vi "Text Format Definition Dialog.vi"(8 "Error In":errorcluster) -> (0 "Error Out":errorcluster, 1 "Result":T1, 2 "Theme Name":string, 3 "Notebook Theme":T2 {"[Named Text Styles]"."Text Formatting"."Font Size" min=6.0 step=1.0})   [LabVIEW 2021, in "Notebook.lvlib"]
doc: "Define text format for different styles"
uses:
  Notebook.lvlib
  Rich Text Box/Text Format List.ctl
  Rich Text Box/Text Colors.ctl
  Notebook Theme.ctl
  Rich Text Box/Named Text Style.ctl
  Rich Text Box/Text Formatting.ctl
  Rich Text Box/Text Style.ctl
  Rich Text Box/Text Alignment.ctl
  Notebook Theme Edit Result.ctl
  Notebook Parameters List.ctl
  Variant/Variant to Data/Variant to String.vi
  Rich Text Box/Rich Text Box.lvlib
  System.Windows.Forms
  Variant/Variant to Data/Variant to Data.lvlib
panel:
  in  "Close":bool
  in  "Mark for Deletion":bool
  in  "Theme Name":string
  in  "Use Font Size for all Styles":bool
  in  "Use Alignment for all Styles":bool
  in  "Use Style for all Styles":bool
  in  "Use Background Color for all Styles":bool
  in  "Use Text Color for all Styles":bool
  in  "Use Font for all Styles":bool
  in  "Cancel":bool
  in  "Apply":bool
  in  "Page Color":T5=enum."White"
  in  "Text Style":T8
  in  "Example Content":refnum<k24>(container) caption="Text Example"
  in  "Text Formatting":T9={"Font"=0, "Text Color"=enum."Unchanged", "Background Color"=enum."Unchanged", "Style"=enum."Regular", "Font Size"=6.0, "Alignment"=enum."Left"} {"Font Size" min=6.0 step=1.0; "Font" items=["Adobe Devanagari", "Agency FB", "Algerian", "Arial", "Arial Black", "Arial Narrow", "Arial Rounded MT Bold", "Bahnschrift", "Bahnschrift Condensed", "Bahnschrift Light", "Bahnschrift Light Condensed", "Bahnschrift Light SemiCondensed", "Bahnschrift SemiBold", "Bahnschrift SemiBold Condensed", "Bahnschrift SemiBold SemiConden", "Bahnschrift SemiCondensed", "Bahnschrift SemiLight", "Bahnschrift SemiLight Condensed", "Bahnschrift SemiLight SemiConde", "Barlow Condensed", "Barlow Condensed Black", "Barlow Condensed ExtraBold", "Barlow Condensed ExtraLight", "Barlow Condensed Light", "Barlow Condensed Medium", "Barlow Condensed SemiBold", "Barlow Condensed Thin", "Baskerville Old Face", "Bauhaus 93", "Bell MT", "Berlin Sans FB", "Berlin Sans FB Demi", "Bernard MT Condensed", "Blackadder ITC", "Bodoni MT", "Bodoni MT Black", "Bodoni MT Condensed", "Bodoni MT Poster Compressed", "Book Antiqua", "Bookman Old Style", "Bookshelf Symbol 7", "Bradley Hand ITC", "Britannic Bold", "Broadway", "Brush Script MT", "Calibri", "Calibri Light", "Californian FB", "Calisto MT", "Cambria", "Cambria Math", "Candara", "Candara Light", "Cascadia Code", "Cascadia Code ExtraLight", "Cascadia Code Light", "Cascadia Code SemiBold", "Cascadia Code SemiLight", "Cascadia Mono", "Cascadia Mono ExtraLight", "Cascadia Mono Light", "Cascadia Mono SemiBold", "Cascadia Mono SemiLight", "Castellar", "Caveat", "Centaur", "Century", "Century Gothic", "Century Schoolbook", "Chiller", "Colonna MT", "Comic Sans MS", "Consolas", "Constantia", "Cooper Black", "Copperplate Gothic Bold", "Copperplate Gothic Light", "Corbel", "Corbel Light", "Cormorant Infant", "Cormorant Infant Light", "Cormorant Infant Medium", "Cormorant Infant SemiBold", "Courier New", "Curlz MT", "Dosis", "Dubai", "Dubai Light", "Dubai Medium", "Ebrima", "Edwardian Script ITC", "Elephant", "Engravers MT", "Eras Bold ITC", "Eras Demi ITC", "Eras Light ITC", "Eras Medium ITC", "Euclid", "Euclid Extra", "Euclid Fraktur", "Euclid Math One", "Euclid Math Two", "Euclid Symbol", "Felix Titling", "Fences", "Footlight MT Light", "Forte", "Franklin Gothic Book", "Franklin Gothic Demi", "Franklin Gothic Demi Cond", "Franklin Gothic Heavy", "Franklin Gothic Medium", "Franklin Gothic Medium Cond", "Freestyle Script", "French Script MT", "Gabriola", "Gadugi", "Garamond", "Georgia", "Gigi", "Gill Sans MT", "Gill Sans MT Condensed", "Gill Sans MT Ext Condensed Bold", "Gill Sans Ultra Bold", "Gill Sans Ultra Bold Condensed", "Gloucester MT Extra Condensed", "Goudy Old Style", "Goudy Stout", "Haettenschweiler", "Harlow Solid Italic", "Harrington", "High Tower Text", "HoloLens MDL2 Assets", "HYSWLongFangSong", "Impact", "Imprint MT Shadow", "Informal Roman", "Ink Free", "Javanese Text", "Jokerman", "Juice ITC", "Kristen ITC", "Kunstler Script", "Lato", "Lato Black", "Lato Hairline", "Lato Light", "Leelawadee", "Leelawadee UI", "Leelawadee UI Semilight", "Lucida Bright", "Lucida Calligraphy", "Lucida Console", "Lucida Fax", "Lucida Handwriting", "Lucida Sans", "Lucida Sans Typewriter", "Lucida Sans Unicode", "Magneto", "Maiandra GD", "Malgun Gothic", "Malgun Gothic Semilight", "Marlett", "Matura MT Script Capitals", "Microsoft Himalaya", "Microsoft JhengHei", "Microsoft JhengHei Light", "Microsoft JhengHei UI", "Microsoft JhengHei UI Light", "Microsoft New Tai Lue", "Microsoft PhagsPa", "Microsoft Sans Serif", "Microsoft Tai Le", "Microsoft Uighur", "Microsoft YaHei", "Microsoft YaHei Light", "Microsoft YaHei UI", "Microsoft YaHei UI Light", "Microsoft Yi Baiti", "MingLiU-ExtB", "MingLiU_HKSCS-ExtB", "Mistral", "Modern No. 20", "Mongolian Baiti", "Monotype Corsiva", "Montserrat", "Montserrat Black", "Montserrat ExtraBold", "Montserrat ExtraLight", "Montserrat Light", "Montserrat Medium", "Montserrat SemiBold", "Montserrat Thin", "MS Gothic", "MS Outlook", "MS PGothic", "MS Reference Sans Serif", "MS Reference Specialty", "MS UI Gothic", "MT Extra", "MT Extra Tiger", "MV Boli", "Myanmar Text", "Niagara Engraved", "Niagara Solid", "Nirmala UI", "Nirmala UI Semilight", "Noto Sans", "Noto Serif", "NSimSun", "OCR A Extended", "Old English Text MT", "Onyx", "Open Sans", "Open Sans ExtraBold", "Open Sans Light", "Open Sans SemiBold", "Origin", "Oswald", "Oswald ExtraLight", "Oswald Light", "Oswald Medium", "Oswald SemiBold", "Palace Script MT", "Palatino Linotype", "Papyrus", "Parchment", "Perpetua", "Perpetua Titling MT", "Playbill", "PMingLiU-ExtB", "Poor Richard", "Pristina", "Rage Italic", "Raleway", "Raleway Black", "Raleway ExtraBold", "Raleway ExtraLight", "Raleway Light", "Raleway Medium", "Raleway SemiBold", "Raleway Thin", "Ravie", "Roboto", "Roboto Black", "Roboto Condensed", "Roboto Condensed Light", "Roboto Light", "Roboto Medium", "Roboto Slab", "Roboto Slab Black", "Roboto Slab Light", "Roboto Slab Medium", "Roboto Slab Thin", "Roboto Thin", "Rockwell", "Rockwell Condensed", "Rockwell Extra Bold", "Script MT Bold", "Segoe MDL2 Assets", "Segoe Print", "Segoe Script", "Segoe UI", "Segoe UI Black", "Segoe UI Emoji", "Segoe UI Historic", "Segoe UI Light", "Segoe UI Semibold", "Segoe UI Semilight", "Segoe UI Symbol", "Showcard Gothic", "SimSun", "SimSun-ExtB", "SimSun-ExtG", "Sitka Banner", "Sitka Display", "Sitka Heading", "Sitka Small", "Sitka Subheading", "Sitka Text", "Snap ITC", "Source Code Pro", "Source Code Pro Black", "Source Code Pro ExtraLight", "Source Code Pro Light", "Source Code Pro Semibold", "Source Sans Pro", "Source Sans Pro Black", "Source Sans Pro ExtraLight", "Source Sans Pro Light", "Source Sans Pro SemiBold", "Stencil", "Sylfaen", "Symbol", "Symbol Tiger", "Symbol Tiger Expert", "Tahoma", "Tempus Sans ITC", "Tiger", "Tiger Expert", "Times New Roman", "Trebuchet MS", "Tw Cen MT", "Tw Cen MT Condensed", "Tw Cen MT Condensed Extra Bold", "Univers-CondBoldOblique", "Univers-Condensed", "Univers-CondensedBold", "UniversCond", "UniversCondBold", "UniversCondLight", "UniversCondLightOblique", "UniversCondOblique", "Verdana", "Viner Hand ITC", "Vivaldi", "Vladimir Script", "Webdings", "Wide Latin", "Wingdings", "Wingdings 2", "Wingdings 3", "Yu Gothic", "Yu Gothic Light", "Yu Gothic Medium", "Yu Gothic UI", "Yu Gothic UI Light", "Yu Gothic UI Semibold", "Yu Gothic UI Semilight", "Zilla Slab", "Zilla Slab Light", "Zilla Slab Medium", "Zilla Slab SemiBold", "ZWAdobeF"]}
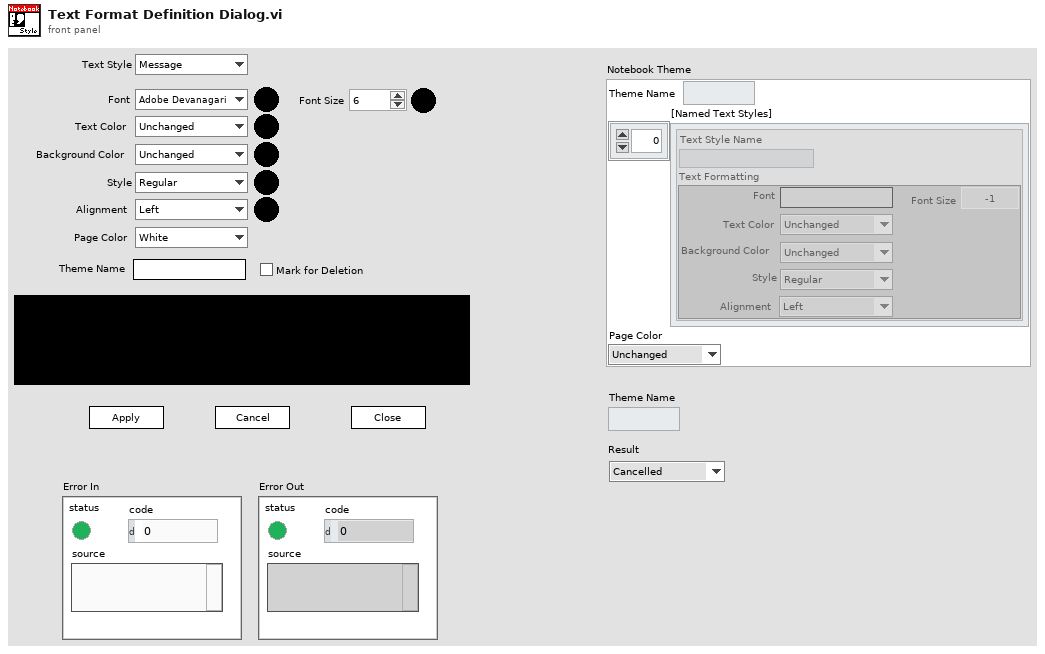
[diagram p1: front panel]
types:
  T1 = typedef "Notebook.lvlib/Notebook Theme Edit Result.ctl" = enum16{"Cancelled", "Modified Theme", "New Theme", "Remove Theme"}
  T2 = typedef "Notebook.lvlib/Notebook Theme.ctl" = cluster{"Theme Name":string, "[Named Text Styles]":T3[], "Page Color":T5}
  T3 = typedef "Notebook.lvlib/Named Text Style.ctl" = cluster{"Text Formatting":T4, "Text Style Name":string}
  T4 = typedef "Rich Text Box.lvlib/Text Formatting.ctl" = cluster{"Font":string, "Text Color":T5, "Background Color":T5, "Style":T6, "Font Size":dbl, "Alignment":T7}
  T5 = typedef "Rich Text Box.lvlib/Text Colors.ctl" = enum16{"Unchanged", "Black", "Blue", "Cyan", "Maroon", "Gray", "Violet", "Green", "Light Green", "Orange", "Yellow", "Magenta", "Red", "White"}
  T6 = typedef "Rich Text Box.lvlib/Text Style.ctl" = enum16{"Regular", "Bold", "Italic", "Underline", "Strikeout"}
  T7 = typedef "Rich Text Box.lvlib/Text Alignment.ctl" = enum16{"Left", "Right", "Center"}
  T8 = typedef "Notebook.lvlib/Text Format List.ctl" = enum16{"Message", "Result", "Error", "Setting", "Verbose", "Warning"}
  T9 = cluster{"Font":u16, "Text Color":T5, "Background Color":T5, "Style":T6, "Font Size":dbl, "Alignment":T7}
  T10 = typedef "Notebook.lvlib/Notebook Parameters List.ctl" = enum16{"First Opening?", "Saved Notebook?", "Saved Notebook Path", "Beep on Error?", "Notebook Themes", "Current Theme Name"}
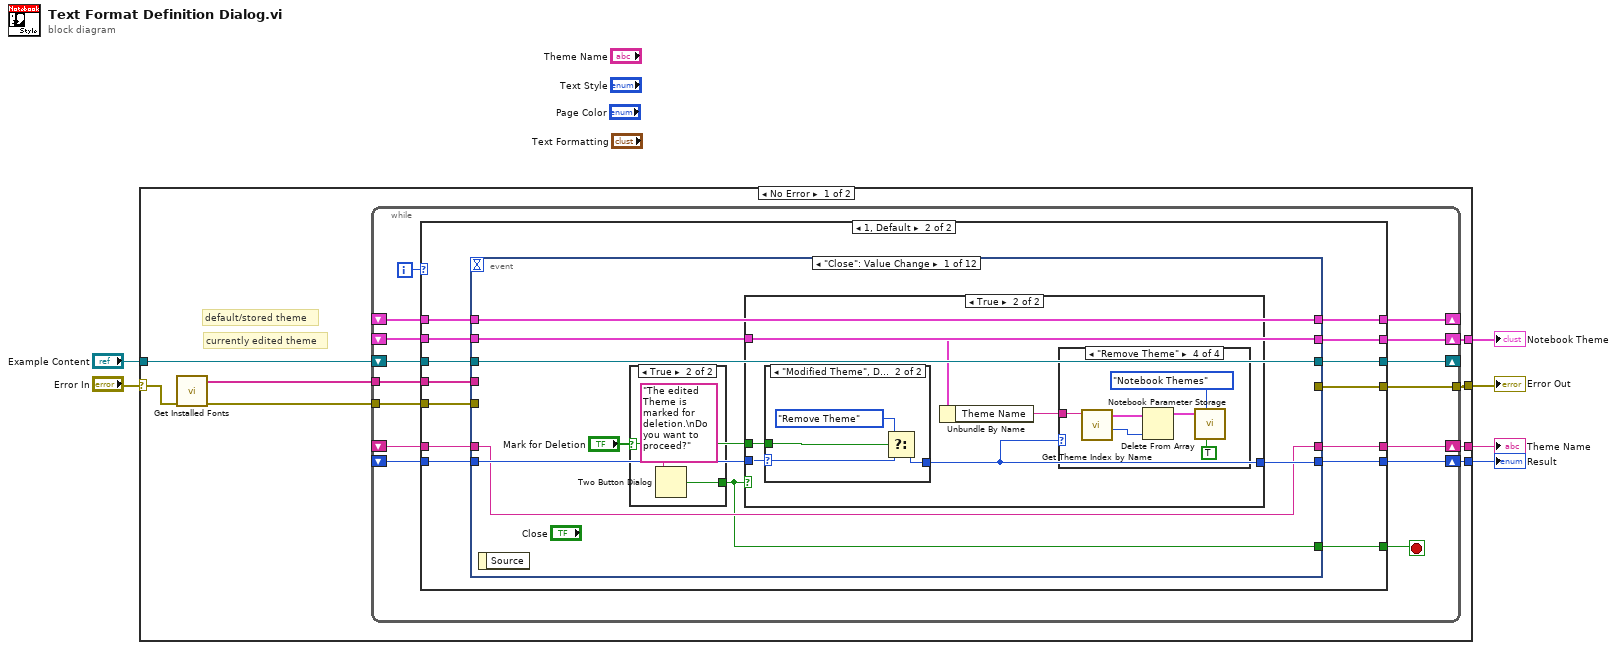
[diagram p0: block diagram]
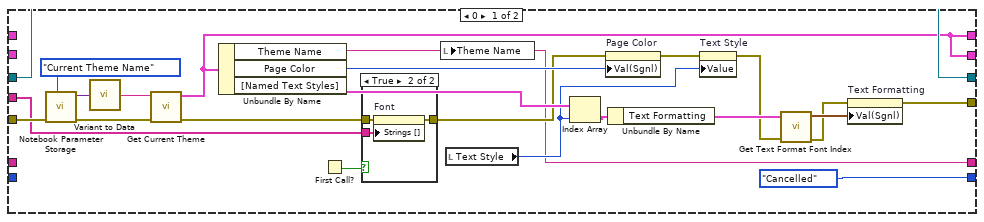
[diagram p2: hidden frame]
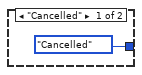
[diagram p8: hidden frame]
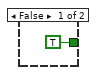
[diagram p9: hidden frame]
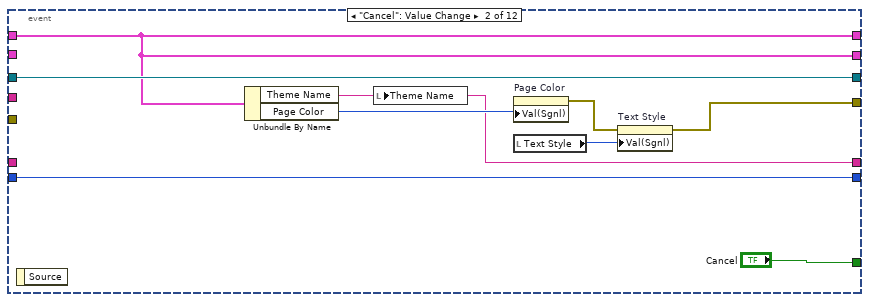
[diagram p10: hidden frame]
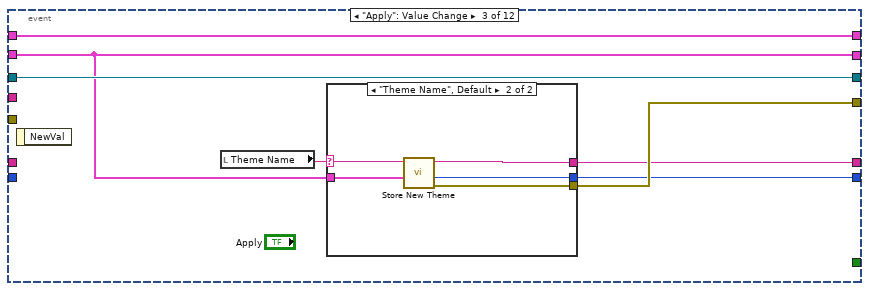
[diagram p11: hidden frame]
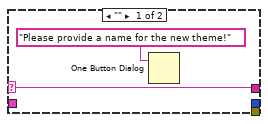
[diagram p12: hidden frame]
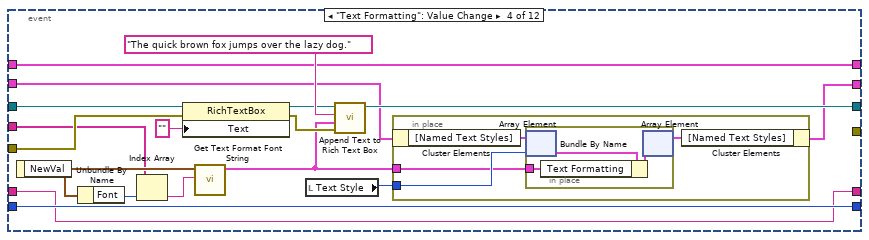
[diagram p13: hidden frame]
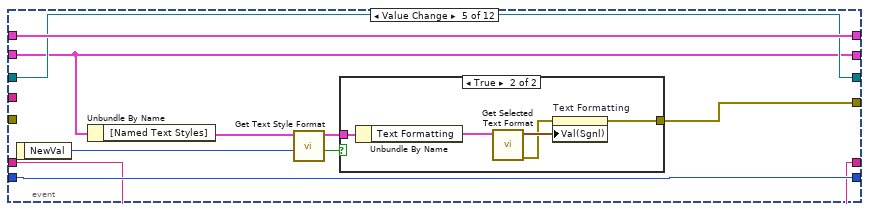
[diagram p14: hidden frame]
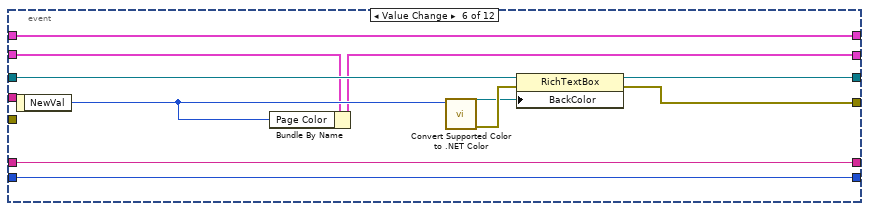
[diagram p16: hidden frame]
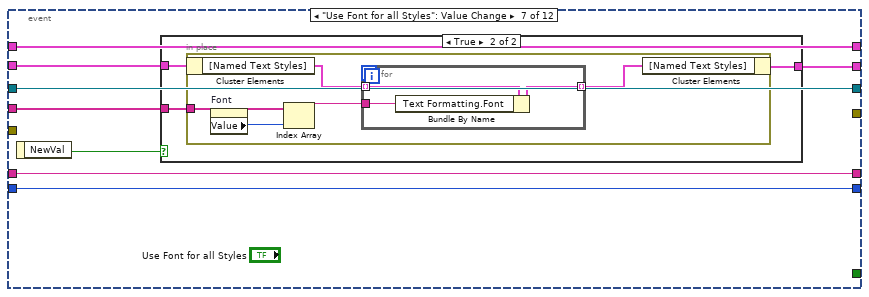
[diagram p17: hidden frame]
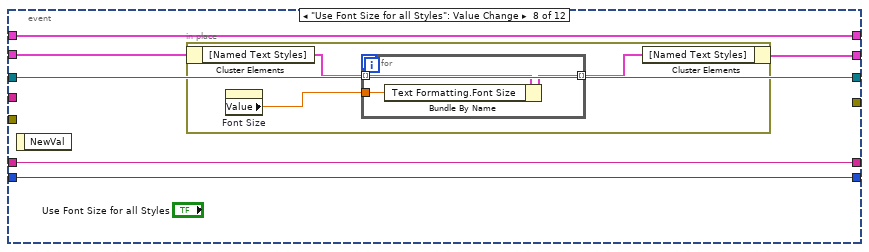
[diagram p19: hidden frame]
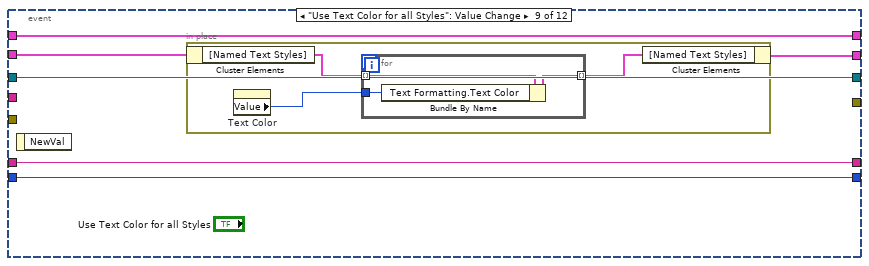
[diagram p20: hidden frame]
diagram:
  n1 = case shown="No Error" "Error In" {
    selector: "Error In" -> [w10 w253]
    tunnel: "Example Content" -> [w13 _]
    tunnel: [w12 _] -> w3
    tunnel: [w11 w253] -> w5
    tunnel: [w8 _] -> w2
    tunnel: [w7 _] -> w1
    frame No Error {
      # "currently edited theme"
      # "default/stored theme"
      n2 = call "Get Installed Fonts.vi"("Error In"=w10) -> ("Error Out"=w9:errorcluster, "Installed Fonts"=w14:string[])  [unwired: 8 in, 1 out]
      n3 = while {
        tunnel: w9 -> [w21]
        tunnel: w14 -> [w28]
        shift-right: [w26] -> _
        shift-left: w13 -> [w27]
        shift-right: [w25] -> _
        shift-left: _ -> [w24]
        tunnel: [w22] -> w11
        shift-right: [w23] -> w12
        shift-left: _ -> [w20]
        shift-right: [w18] -> w8
        shift-left: _ -> [w16]
        shift-right: [w17] -> w7
        shift-left: _ -> [w15]
        i -> [w19]
        stop <- w29 stop-if-true
        n4 = case shown="1, Default" w19 {
          tunnel: [_ w70] -> w29
          tunnel: w28 -> [w49 w69]
          tunnel: w27 -> [w52 w68]
          tunnel: [w52 w67] -> w26
          tunnel: [w45 w66] -> w22
          tunnel: [w47 w64] -> w25
          tunnel: w24 -> [_ w65]
          tunnel: [w47 w63] -> w23
          tunnel: w21 -> [w51 w61]
          tunnel: w20 -> [_ w62]
          tunnel: [Notebook_Theme_Edit_Result."Cancelled" ("Result") w60] -> w18
          tunnel: [w32 w59] -> w17
          tunnel: w16 -> [_ w58]
          tunnel: w15 -> [_ w57]
          frame 0 {
            n5 = call "Notebook Parameter Storage.vi"("Notebook Parameter List"=Notebook_Parameters_List."Current Theme Name", "Error In"=w51) -> ("Error Out"=w35:errorcluster, "Data out"=w38:variant)  [unwired: 8 in]
            n6 = call-poly "Variant to Data.vi"("Variant"=w38) -> ("String"=w36:string)  [unwired: 8 in]
            n7 = call "Get Current Theme.vi"("Error In"=w35, "Theme Name"=w36) -> ("Error Out"=w50:errorcluster, "Notebook Theme"=w47:T2)  [unwired: 7 in, 1 out]
            n8 = Unbundle By Name(w47) -> ("Theme Name"=w32:string, "Page Color"=w46:T5, "[Named Text Styles]"=w44:T3[])
            n9 = First Call?() -> (First Call?: T/F=w30:bool)
            n10 = case shown="True" w30 {
              tunnel: w50 -> [w53 w56]
              tunnel: w49 -> [_ w55]
              tunnel: [w53 w54] -> w40
              frame False {
              }
              frame True {
                n11 = property on="Font" class="Ring (strict)"(error in=w56, "Strings []"=w55) -> (error out=w54:errorcluster)  [unwired: 1 in, 1 out]
              }
            }
            n12 = local write "Theme Name"(w32) -> ()
            n13 = local read "Text Style"() -> (w34:T8)
            n14 = Index Array(array=w44, index=w34) -> (element=w43:T3)
            n15 = property on="Page Color" class="Enum (strict)"(error in=w40, "Val(Sgnl)"=w46) -> (error out=w48:errorcluster)  [unwired: 1 in, 1 out]
            n16 = Unbundle By Name(w43) -> ("Text Formatting"=w42:T4)
            n17 = property on="Text Style" class="Enum (strict)"(error in=w48, "Value"=w34) -> (error out=w33:errorcluster)  [unwired: 1 in, 1 out]
            n18 = call "Get Text Format Font Index.vi"("Error In"=w33, "Text Format"=w42) -> ("Error Out"=w39:errorcluster, "Text Format Dialog"=w41:T9)  [unwired: 8 in]
            n19 = property on="Text Formatting" class="Clust (strict)"(error in=w39, "Val(Sgnl)"=w41) -> (error out=w45:errorcluster)  [unwired: 1 in, 1 out]
          }
          frame 1, Default {
            n20 = event shown="[0] \"Close\": Value Change" {
              selector: _ -> [_ _ _ _ _ _ _ _ _ _ _ _]
              dyn-events: _ -> [_ _ _ _ _ _ _ _ _ _ _ _]
              timeout: _ -> [_ _ _ _ _ _ _ _ _ _ _ _]
              tunnel: [w71 "Cancel" _ _ _ _ _ _ _ _ _ _] -> w70
              tunnel: w69 -> [_ _ _ w123 _ _ w173 _ _ _ _ _]
              tunnel: w68 -> [w78 w106 w113 w135 w155 w170 w180 w198 w210 w222 w234 w246]
              tunnel: [w78 w106 w113 w134 w155 w169 w180 w198 w210 w222 w234 w246] -> w67
              tunnel: [_ w101 w110 _ w152 w168 _ _ _ _ _ _] -> w66
              tunnel: w65 -> [w77 w104 w114 w130 w156 w167 w179 w197 w209 w221 w233 w245]
              tunnel: [w77 w104 w114 w130 w156 w167 w179 w197 w209 w221 w233 w245] -> w64
              tunnel: [w74 w104 w111 w129 w151 w164 w175 w193 w205 w217 w229 w241] -> w63
              tunnel: w62 -> [w74 _ w111 w128 w151 w165 w176 w194 w206 w218 w230 w242]
              tunnel: w61 -> [_ _ _ w133 _ _ _ _ _ _ _ _]
              tunnel: [w75 w99 w109 w127 w148 w163 w178 w196 w208 w220 w232 w244] -> w60
              tunnel: [w73 w100 w108 w126 w147 w162 w177 w195 w207 w219 w231 w243] -> w59
              tunnel: w58 -> [w76 w99 _ w127 w148 w163 w178 w196 w208 w220 w232 w244]
              tunnel: w57 -> [w73 _ _ w126 w147 w162 w177 w195 w207 w219 w231 w243]
              event "Close": Value Change {
                n21 = event-data() -> ()  [unwired: 1 in, 1 out]
                n22 = case shown="True" "Mark for Deletion" {
                  tunnel: [TRUE ("T button?") w97] -> w71
                  frame False {
                  }
                  frame True {
                    n23 = Two Button Dialog(message="The edited Theme is marked for deletion.\nDo you want to proceed?") -> (T button?=w97:bool)  [unwired: 2 in]
                  }
                }
                n24 = case shown="True" w71 {
                  tunnel: w76 -> [w79 w84]
                  tunnel: [w79 w83] -> w75
                  tunnel: w74 -> [_ w82]
                  tunnel: "Mark for Deletion" -> [_ w80]
                  frame False {
                  }
                  frame True {
                    n25 = case shown="\"Modified Theme\", Default" w84 {
                      selector: w84 -> [_ w94]
                      tunnel: [Notebook_Theme_Edit_Result."Cancelled" ("Result") w93] -> w83
                      tunnel: w80 -> [_ w92]
                      frame "Cancelled" {
                      }
                      frame "Modified Theme", Default {
                        n26 = Select(t=Notebook_Theme_Edit_Result."Remove Theme" ("Result"), s=w92, f=w94) -> (s? t:f=w93:T1)
                      }
                    }
                    n27 = Unbundle By Name(w82) -> ("Theme Name"=w81:string)
                    n28 = case shown="\"Remove Theme\"" w83 {
                      tunnel: w81 -> [_ _ _ w90]
                      frame "Cancelled", Default {
                      }
                      frame "Modified Theme" {
                      }
                      frame "New Theme" {
                      }
                      frame "Remove Theme" {
                        n29 = call "Get Theme Index by Name.vi"("Theme Name"=w90) -> ("Theme Index"=w86:i32, "Theme Array"=w87:T2[])  [unwired: 7 in, 2 out]
                        n30 = Delete From Array(array=w87, index=w86) -> (array with subset deleted=w88:T2[])  [unwired: 1 in, 1 out]
                        n31 = call "Notebook Parameter Storage.vi"("Get(F)/Set"=TRUE, "Notebook Parameter List"=Notebook_Parameters_List."Notebook Themes", "Data in"=w88) -> ()  [unwired: 7 in, 2 out]
                      }
                    }
                  }
                }
              }
              event "Cancel": Value Change {
                n32 = event-data() -> ()  [unwired: 1 in, 1 out]
                n33 = Unbundle By Name(w104) -> ("Theme Name"=w100:string, "Page Color"=w103:T5)
                n34 = local write "Theme Name"(w100) -> ()
                n35 = property on="Page Color" class="Enum (strict)"("Val(Sgnl)"=w103) -> (error out=w102:errorcluster)  [unwired: 2 in, 1 out]
                n36 = local read "Text Style"() -> (w105:T8)
                n37 = property on="Text Style" class="Enum (strict)"(error in=w102, "Val(Sgnl)"=w105) -> (error out=w101:errorcluster)  [unwired: 1 in, 1 out]
              }
              event "Apply": Value Change {
                n38 = event-data() -> ()  [unwired: 1 in, 1 out]
                n39 = local read "Theme Name"() -> (w112:string)
                n40 = case shown="\"Theme Name\", Default" w112 {
                  selector: w112 -> [w115 w121]
                  tunnel: w111 -> [_ w120]
                  tunnel: [_ w119] -> w110
                  tunnel: [_ w118] -> w109
                  tunnel: [w115 w117] -> w108
                  frame "" {
                    n41 = One Button Dialog(message="Please provide a name for the new theme!") -> ()  [unwired: 1 in, 1 out]
                  }
                  frame "Theme Name", Default {
                    n42 = call "Store New Theme.vi"("Notebook Theme"=w120, "New Theme Name"=w121) -> ("Error Out"=w119:errorcluster, "Result"=w118:T1, "New Theme Name (dup)"=w117:string)  [unwired: 7 in]
                  }
                }
              }
              event "Text Formatting": Value Change {
                n43 = event-data() -> ("NewVal"=w125:T9)  [unwired: 1 in]
                n44 = Unbundle By Name(w125) -> ("Font"=w124:u16)
                n45 = Index Array(array=w123, index=w124) -> (element=w122:string)
                n46 = property class="RichTextBox"(reference=w135, error in=w133, "Text"="") -> (reference out=w138:refnum<k24>, error out=w136:errorcluster)
                n47 = call "Get Text Format Font String.vi"("Font Name"=w122, "Text Format Dialog"=w125) -> ("Text Format"=w132:T4)  [unwired: 8 in, 1 out]
                n48 = local read "Text Style"() -> (w131:T8)
                n49 = call "Append Text to Rich Text Box.vi"("error in (no error)"=w136, "Text Formatting"=w132, "String"="The quick brown fox jumps over the lazy dog.", ".NET Refnum in"=w138) -> (".NET Refnum out"=w134:refnum<k24>)  [unwired: 5 in, 2 out]
                n50 = in-place {
                  in-place-border: w131 -> [w143]
                  in-place-border: w132 -> [w142]
                  n51 = in-place-cluster #1(w128) -> ("[Named Text Styles]"=w140:T3[])
                  n52 = in-place {
                    in-place-border: w142 -> [w146]
                    n53 = in-place-array #2(w140, w143) -> (w144:T3)
                    n54 = Bundle By Name(cluster=w144, "Text Formatting"=w146) -> (w145:T3)
                    n55 = in-place-array #2(w145) -> (w141:T3[])  [unwired: 1 out]
                  }
                  n56 = in-place-cluster #1("[Named Text Styles]"=w141) -> (w129:T2)
                }
              }
              event Value Change {
                n57 = event-data() -> ("NewVal"=w153:T8)  [unwired: 1 in]
                n58 = Unbundle By Name(w151) -> ("[Named Text Styles]"=w150:T3[])
                n59 = call "Get Text Style Format.vi"("Style Name"=w153, "[Named Text Styles]"=w150) -> ("Found?"=w149:bool, "Text Style"=w154:T3)  [unwired: 8 in]
                n60 = case shown="True" w149 {
                  tunnel: w154 -> [_ w161]
                  tunnel: [_ w157] -> w152
                  frame False {
                  }
                  frame True {
                    n61 = Unbundle By Name(w161) -> ("Text Formatting"=w160:T4)
                    n62 = call "Get Selected Text Format.vi"("Text Formatting in"=w160) -> ("Error Out"=w158:errorcluster, "Text Formatting"=w159:T9)  [unwired: 9 in]
                    n63 = property on="Text Formatting" class="Clust (strict)"(error in=w158, "Val(Sgnl)"=w159) -> (error out=w157:errorcluster)  [unwired: 1 in, 1 out]
                  }
                }
              }
              event Value Change {
                n64 = event-data() -> ("NewVal"=w166:T5)  [unwired: 1 in]
                n65 = Bundle By Name(cluster=w165, "Page Color"=w166) -> (w164:T2)
                n66 = call "Convert Supported Color to .NET Color.vi"("Text Color"=w166) -> ("error out"=w172:errorcluster, ".NET Color"=w171:refnum<k24>)  [unwired: 9 in]
                n67 = property class="RichTextBox"(reference=w170, error in=w172, "BackColor"=w171) -> (reference out=w169:refnum<k24>, error out=w168:errorcluster)
              }
              event "Use Font for all Styles": Value Change {
                n68 = event-data() -> ("NewVal"=w174:bool)  [unwired: 1 in]
                n69 = case shown="True" w174 {
                  tunnel: w176 -> [w181 w184]
                  tunnel: [w181 w183] -> w175
                  tunnel: w173 -> [_ w182]
                  frame False {
                  }
                  frame True {
                    n70 = in-place {
                      in-place-border: w182 -> [w187]
                      n71 = in-place-cluster #3(w184) -> ("[Named Text Styles]"=w189:T3[])
                      n72 = property on="Font" class="Ring (strict)"() -> ("Value"=w186:u16)  [unwired: 2 in, 2 out]
                      n73 = Index Array(array=w187, index=w186) -> (element=w185:string)
                      n74 = for {
                        tunnel: w185 -> [w192]
                        tunnel: w189 -> [w191] mode=indexing
                        tunnel: [w190] -> w188 mode=indexing
                        n75 = Bundle By Name(cluster=w191, "Text Formatting.Font"=w192) -> (w190:T3)
                      }
                      n76 = in-place-cluster #3("[Named Text Styles]"=w188) -> (w183:T2)
                    }
                  }
                }
              }
              event "Use Font Size for all Styles": Value Change {
                n77 = event-data() -> ()  [unwired: 1 in, 1 out]
                n78 = in-place {
                  n79 = in-place-cluster #4(w194) -> ("[Named Text Styles]"=w201:T3[])
                  n80 = property on="Font Size" class="DigNum (strict)"() -> ("Value"=w199:dbl)  [unwired: 2 in, 2 out]
                  n81 = for {
                    tunnel: w199 -> [w204]
                    tunnel: w201 -> [w203] mode=indexing
                    tunnel: [w202] -> w200 mode=indexing
                    n82 = Bundle By Name(cluster=w203, "Text Formatting.Font Size"=w204) -> (w202:T3)
                  }
                  n83 = in-place-cluster #4("[Named Text Styles]"=w200) -> (w193:T2)
                }
              }
              event "Use Text Color for all Styles": Value Change {
                n84 = event-data() -> ()  [unwired: 1 in, 1 out]
                n85 = in-place {
                  n86 = in-place-cluster #5(w206) -> ("[Named Text Styles]"=w213:T3[])
                  n87 = property on="Text Color" class="Enum (strict)"() -> ("Value"=w211:T5)  [unwired: 2 in, 2 out]
                  n88 = for {
                    tunnel: w211 -> [w216]
                    tunnel: w213 -> [w215] mode=indexing
                    tunnel: [w214] -> w212 mode=indexing
                    n89 = Bundle By Name(cluster=w215, "Text Formatting.Text Color"=w216) -> (w214:T3)
                  }
                  n90 = in-place-cluster #5("[Named Text Styles]"=w212) -> (w205:T2)
                }
              }
              event "Use Background Color for all Styles": Value Change {
                n91 = event-data() -> ()  [unwired: 1 in, 1 out]
                n92 = in-place {
                  n93 = in-place-cluster #6(w218) -> ("[Named Text Styles]"=w225:T3[])
                  n94 = property on="Background Color" class="Enum (strict)"() -> ("Value"=w223:T5)  [unwired: 2 in, 2 out]
                  n95 = for {
                    tunnel: w223 -> [w228]
                    tunnel: w225 -> [w227] mode=indexing
                    tunnel: [w226] -> w224 mode=indexing
                    n96 = Bundle By Name(cluster=w227, "Text Formatting.Background Color"=w228) -> (w226:T3)
                  }
                  n97 = in-place-cluster #6("[Named Text Styles]"=w224) -> (w217:T2)
                }
              }
              event "Use Style for all Styles": Value Change {
                n98 = event-data() -> ()  [unwired: 1 in, 1 out]
                n99 = in-place {
                  n100 = in-place-cluster #7(w230) -> ("[Named Text Styles]"=w237:T3[])
                  n101 = property on="Style" class="Enum (strict)"() -> ("Value"=w235:T6)  [unwired: 2 in, 2 out]
                  n102 = for {
                    tunnel: w235 -> [w240]
                    tunnel: w237 -> [w239] mode=indexing
                    tunnel: [w238] -> w236 mode=indexing
                    n103 = Bundle By Name(cluster=w239, "Text Formatting.Style"=w240) -> (w238:T3)
                  }
                  n104 = in-place-cluster #7("[Named Text Styles]"=w236) -> (w229:T2)
                }
              }
              event "Use Alignment for all Styles": Value Change {
                n105 = event-data() -> ()  [unwired: 1 in, 1 out]
                n106 = in-place {
                  n107 = in-place-cluster #8(w242) -> ("[Named Text Styles]"=w249:T3[])
                  n108 = property on="Alignment" class="Enum (strict)"() -> ("Value"=w247:T7)  [unwired: 2 in, 2 out]
                  n109 = for {
                    tunnel: w247 -> [w252]
                    tunnel: w249 -> [w251] mode=indexing
                    tunnel: [w250] -> w248 mode=indexing
                    n110 = Bundle By Name(cluster=w251, "Text Formatting.Alignment"=w252) -> (w250:T3)
                  }
                  n111 = in-place-cluster #8("[Named Text Styles]"=w248) -> (w241:T2)
                }
              }
            }
          }
        }
      }
    }
    frame Error {
    }
  }
  "Notebook Theme" <- w3
  "Error Out" <- w5
  "Result" <- w2
  "Theme Name" <- w1
